vi "Timestamp To ISO String.vi"(8 "error in (no error)":errorcluster, 10 "Universal time (F)":bool, 11 "Timestamp":timestamp) -> (0 "error out":errorcluster, 3 "ISO Timestamp String":string)   [LabVIEW 2019, in "JKI JSON Serialization.lvlib" / "JSON Serializer.lvclass"]
doc: "Converts LabVIEW timestamp to ISO formatted timestamp string.\n\nJKI JSON 1.1.10.37\nTomi Maila - JKI\nCopyright (c) 2017, JKI"
uses:
  JSON Serializer.lvclass
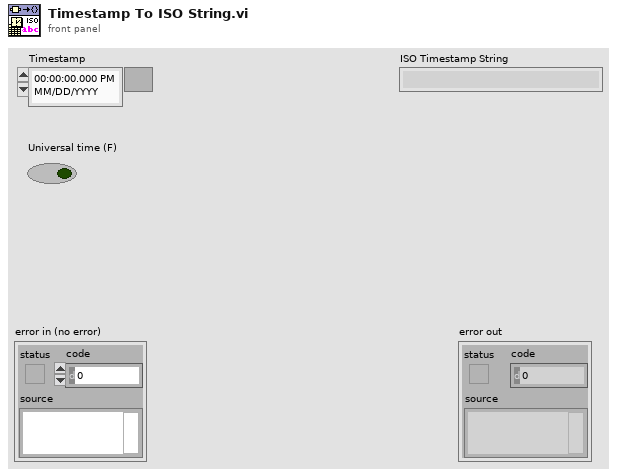
[diagram p1: front panel]
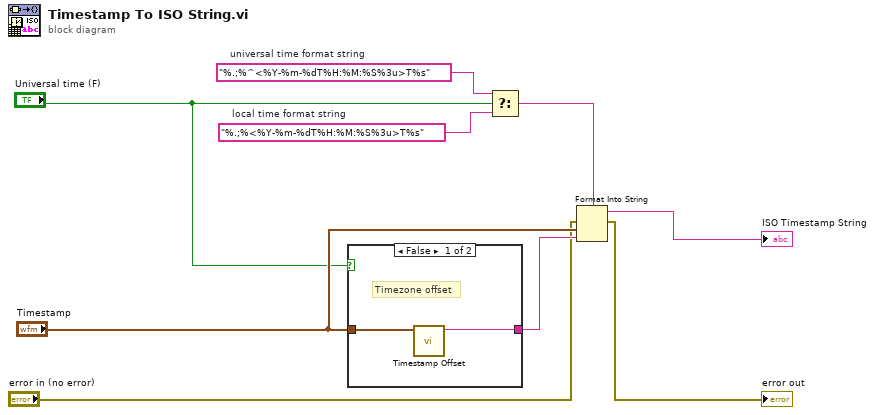
[diagram p0: block diagram]
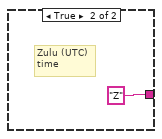
[diagram p2: hidden frame]
diagram:
  w8 = "%.;%<%Y-%m-%dT%H:%M:%S%3u>T%s"  # local time format string
  w9 = "%.;%^<%Y-%m-%dT%H:%M:%S%3u>T%s"  # universal time format string
  n1 = case shown="False" "Universal time (F)" {
    tunnel: "Timestamp" -> [w11 _]
    tunnel: [w10 "Z"] -> w7
    frame False {
      # "Timezone offset"
      n2 = call "Timestamp Offset.vi"("Timestamp"=w11) -> ("Timezone offset string"=w10:string)  [unwired: 10 in]
    }
    frame True {
      # "Zulu (UTC)\ntime"
    }
  }
  n3 = Select(t=w9, s="Universal time (F)", f=w8) -> (s? t:f=w6:string)
  n4 = Format Into String(format string=w6, error in="error in (no error)", "Timestamp", w7) -> (resulting string=→"ISO Timestamp String":string, error out=→"error out":errorcluster)  [unwired: 1 in]
